vi "MergeDirectoriesAndDeleteOld.vi"(7 "Delete Source? (FALSE)":bool, 8 "error in (no error)":errorcluster, 10 "target directory path":path, 11 "source directory path":path) -> (0 "error out":errorcluster, 3 "dup target directory path":path)   [LabVIEW 2024, in "openg_file.lvlib"]
doc: "Copies the contents of source directory into the destination directory. If source directory has subdirectories they will be copied into the destination directory recursively. Optionally, existing files may be overwritten, by setting the \"Overwrite Existing Files?\" input to TRUE. If you attempt to overwrite an existing file without setting to TRUE ans error will be returned. If FALSE, existing files will not be overwritten and no error wil be returned, Optionally, read-only files may be overwritten, by setting the \"Ignore Read-Only?\" input to TRUE. If you attempt to overwrite a read-only files without setting to TRUE an error will be returned. Optionally, by setting the \"Delete Source?\" input to TRUE the source directory will be deleted upon merge completion if no errors occured."
uses:
  <userlib>/_OpenG.lib/file/file.llb/openg_file.lvlib
  <userlib>/_OpenG.lib/file/file.llb/Build Path - File Names Array__ogtk.vi
  <userlib>/_OpenG.lib/file/file.llb/Compare Two Paths - Scalar__ogtk.vi
  <userlib>/_OpenG.lib/file/file.llb/Build Path - Traditional - path__ogtk.vi
  <userlib>/_OpenG.lib/file/file.llb/Strip Path - Traditional__ogtk.vi
panel:
  # "OpenG Library.vi\n\nMerge Directories.vi\n\nCopies the contents of source directory into the destination directory.\n\nPlease visit http://www.OpenG.org to learn about the\nOpen Source LabVIEW software movement.\n\nNOTICE -- YOU MUST LEAVE THIS NOTICE IN PLACE.  PER THE TERMS OF THE LICENSE BELOW, YOU MAY SUBLICENSE THIS SOFTWARE \nIN ANY WAY THAT DOES NOT CONFLICT WITH THIS LICENSE.\n\n### BSD License (http://www.opensource.org/licenses/bsd-license.php) Begin ###\n \nCopyright (c) 2002-2004, Jim Kring <jim@jimkring.com>\nCopyright (c) 2002, Cal-Bay Systems, Inc. <info@calbay.com>\n\nAll rights reserved.\n\nRedistribution and use in source and binary forms, with or without modification, are permitted provided that the following conditions are met:\n\n    * Redistributions of source code must retain the above copyright notice, this list of conditions and the following disclaimer.\n    * Redistributions in binary form must reproduce the above copyright notice, this list of conditions and the following disclaimer in the \n       documentation and/or other materials provided with the distribution.\n    * Neither the name of SciWare, James Kring, Inc., nor the names of its contributors may be used to endorse or promote products derived \n       from this software without specific prior written permission.\n\nTHIS SOFTWARE IS PROVIDED BY THE COPYRIGHT HOLDERS AND CONTRIBUTORS \"AS IS\" AND ANY EXPRESS OR IMPLIED WARRANTIES, \nINCLUDING, BUT NOT LIMITED TO, THE IMPLIED WARRANTIES OF MERCHANTABILITY AND FITNESS FOR A PARTICULAR PURPOSE ARE \nDISCLAIMED. IN NO EVENT SHALL THE COPYRIGHT OWNER OR CONTRIBUTORS BE LIABLE FOR ANY DIRECT, INDIRECT, INCIDENTAL,\n SPECIAL, EXEMPLARY, OR CONSEQUENTIAL DAMAGES (INCLUDING, BUT NOT LIMITED TO, PROCUREMENT OF SUBSTITUTE GOODS OR \nSERVICES; LOSS OF USE, DATA, OR PROFITS; OR BUSINESS INTERRUPTION) HOWEVER CAUSED AND ON ANY THEORY OF LIABILITY, \nWHETHER IN CONTRACT, STRICT LIABILITY, OR TORT (INCLUDING NEGLIGENCE OR OTHERWISE) ARISING IN ANY WAY OUT OF THE USE \nOF THIS SOFTWARE, EVEN IF ADVISED OF THE POSSIBILITY OF SUCH DAMAGE.\n\n### BSD License End ###"
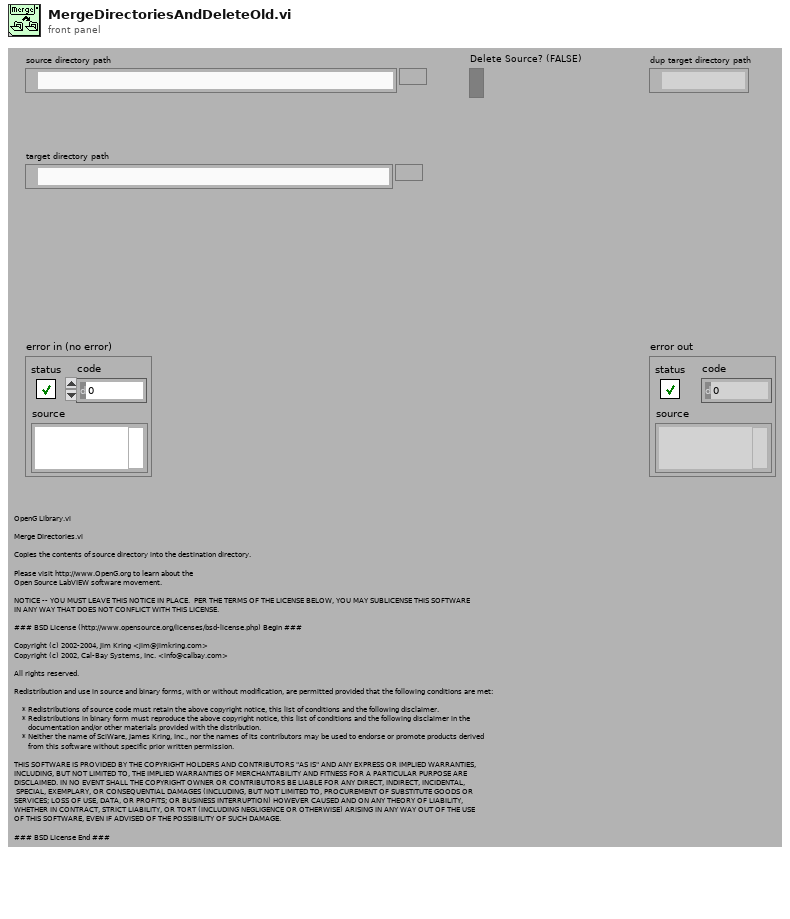
[diagram p1: front panel]
types:
  T1 = cluster{"Archive":bool, "Normal":bool, "Temporary":bool, "Compressed":bool, "Offline":bool, "Content Indexed":bool, "Encrypted (cannot set)":bool}
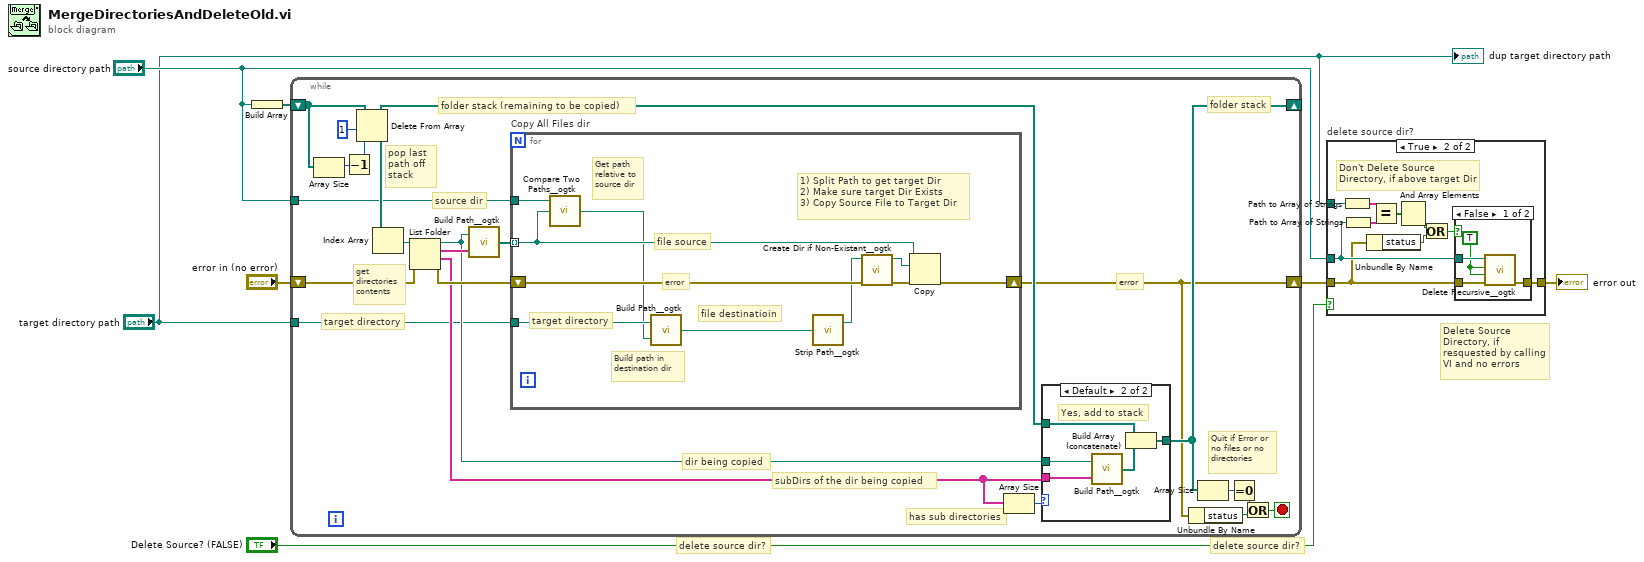
[diagram p0: block diagram]
diagram:
  # "Delete Source Directory, if resquested by calling VI and no errors"
  # "delete source dir?"
  # "delete source dir?"
  n1 = Build Array("source directory path") -> (w7:path[])
  n2 = while {
    shift-right: [w14] -> _
    shift-left: w7 -> [w17]
    shift-right: [w8] -> w5
    shift-left: "error in (no error)" -> [w18]
    tunnel: "source directory path" -> [w10]
    tunnel: "target directory path" -> [w9]
    stop <- w19 stop-if-true
    (unwired) T1 {"Archive"=FALSE, "Normal"=FALSE, "Temporary"=FALSE, "Compressed"=FALSE, "Offline"=FALSE, "Content Indexed"=FALSE, "Encrypted (cannot set)"=FALSE} ("FileAttribute")
    # "folder stack"
    # "error"
    # "target directory"
    # "subDirs of the dir being copied"
    # "dir being copied"
    # "folder stack (remaining to be copied)"
    # "source dir"
    # "get directories contents"
    # "pop last path off stack"
    # "Quit if Error or no files or no directories"
    # "has sub directories"
    n3 = Array Size(array=w17) -> (size(s)=w15:i32)
    n4 = Decrement(x=w15) -> (x-1=w16:i32)
    n5 = Delete From Array(array=w17, length=1 ("Length"), index=w16) -> (deleted portion=w28:path[], array with subset deleted=w23:path[])
    n6 = Index Array(array=w28) -> (element=w27:path)  [unwired: 1 in]
    n7 = List Folder(path=w27, error in=w18) -> (path out=w12:path, filenames=w13:string[], folder names=w24:string[], error out=w26:errorcluster)  [unwired: 2 in]
    n8 = call-poly <userlib>:"Build Path__ogtk.vi"("name or relative path"=w13, "base path"=w12) -> ("appended path"=w11:path[])
    n9 = for "Copy All Files dir" {
      shift-right: [w42] -> w8
      shift-left: w26 -> [w43]
      tunnel: w11 -> [w40] mode=indexing
      tunnel: w10 -> [w41]
      tunnel: w9 -> [w45]
      # "1) Split Path to get target Dir\n2) Make sure target Dir Exists\n3) Copy Source File to Target Dir"
      # "file destinatioin"
      # "file source"
      # "target directory"
      # "error"
      # "Build path in destination dir"
      # "Get path relative to source dir"
      n10 = call-poly <userlib>:"Compare Two Paths__ogtk.vi"("path2"=w40, "path1"=w41) -> ("relative path from 1 to 2"=w39:path)  [unwired: 1 in, 2 out]
      n11 = call-poly <userlib>:"Build Path__ogtk.vi"("name or relative path"=w39, "base path"=w45) -> ("appended path"=w44:path)
      n12 = call-poly <userlib>:"Strip Path__ogtk.vi"("path"=w44) -> ("stripped path"=w36:path)  [unwired: 1 out]
      n13 = call <userlib>:"Create Dir if Non-Existant__ogtk.vi"("error in (no error)"=w43, "Directory Path"=w36) -> ("error out"=w38:errorcluster, "dup Directory Path"=w37:path)  [unwired: 7 in, 1 out]
      n14 = Copy(8:w38, 10:w37, 11:w40) -> (0:w42:errorcluster)  [unwired: 2 in, 2 out]
    }
    n15 = Array Size(array=w24) -> (size(s)=w25:i32)
    n16 = case shown="Default" w25 {
      tunnel: w12 -> [_ w31]
      tunnel: w24 -> [_ w35]
      tunnel: w23 -> [w30 w33]
      tunnel: [w30 w32] -> w14
      frame 0 {
      }
      frame Default {
        # "Yes, add to stack"
        n17 = call-poly <userlib>:"Build Path__ogtk.vi"("name or relative path"=w35, "base path"=w31) -> ("appended path"=w34:path[])
        n18 = Build Array (concatenate)(w33, w34) -> (w32:path[])
      }
    }
    n19 = Unbundle By Name(w8) -> ("status"=w21:bool)
    n20 = Array Size(array=w14) -> (size(s)=w22:i32)
    n21 = Equal To 0?(x=w22) -> (x = 0?=w20:bool)
    n22 = Or(x=w20, y=w21) -> (x .or. y?=w19:bool)
  }
  n23 = case "delete source dir?" shown="True" "Delete Source? (FALSE)" {
    tunnel: w5 -> [w46 w50]
    tunnel: [w46 w56] -> w4
    tunnel: "source directory path" -> [_ w54]
    tunnel: "target directory path" -> [_ w55]
    frame False {
    }
    frame True {
      # "Don't Delete Source Directory, if above target Dir"
      n24 = Path to Array of Strings(0:w55) -> (2:w53:string[])  [unwired: 1 out]
      n25 = Path to Array of Strings(0:w54) -> (2:w52:string[])  [unwired: 1 out]
      n26 = Unbundle By Name(w50) -> ("status"=w47:bool)
      n27 = Equal?(x=w53, y=w52) -> (x = y?=w51:bool[])
      n28 = And Array Elements(Boolean array=w51) -> (logical AND=w49:bool)
      n29 = Or(x=w49, y=w47) -> (x .or. y?=w48:bool)
      n30 = case shown="False" w48 {
        tunnel: w54 -> [w60 _]
        tunnel: [w59 w61] -> w56
        tunnel: w50 -> [w57 w61]
        frame False {
          w58 = TRUE
          n31 = call <userlib>:"Delete Recursive__ogtk.vi"("error in (no error)"=w57, "Ignore Read-Only? (FALSE)"=w58, "Recursive? (FALSE)"=w58, "Path"=w60) -> ("error out"=w59:errorcluster)  [unwired: 6 in, 1 out]
        }
        frame True {
        }
      }
    }
  }
  "error out" <- w4
  "dup target directory path" <- "target directory path"
